vi "LogTracepoint.vi"(8 "error in (no error)":errorcluster, 9 "log string":string, 10 "tracepoint":string, 11 "qbus in":refnum<class "Qbus.lvclass">) -> (0 "error out":errorcluster, 3 "qbus out":refnum<class "Qbus.lvclass">)   [LabVIEW 2017, in "TraceLogger.lvlib"]
doc: "Writes an instance of a tracepoint to a temporary tracelog file on the device disk and sends the instance to NI InsightCM Server to be saved in its tracelog. If the tracepoint is disabled, this VI ignores the input."
uses:
  <vilib>/addons/TraceLogger/TraceLogger.lvlib
  <vilib>/addons/Qbus/Qbus.lvclass
  <vilib>/addons/TraceLogger/controls/LogTracepoint.ctl
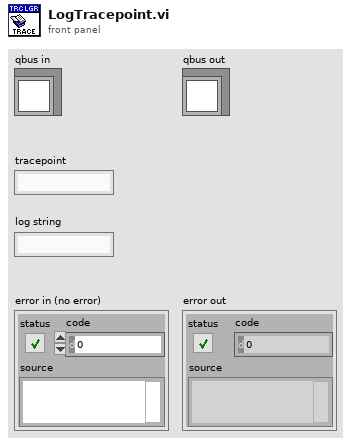
[diagram p1: front panel]
types:
  T1 = typedef "TraceLogger.lvlib/LogTracepoint.ctl" = cluster{"tracepoint":string, "log string":string}
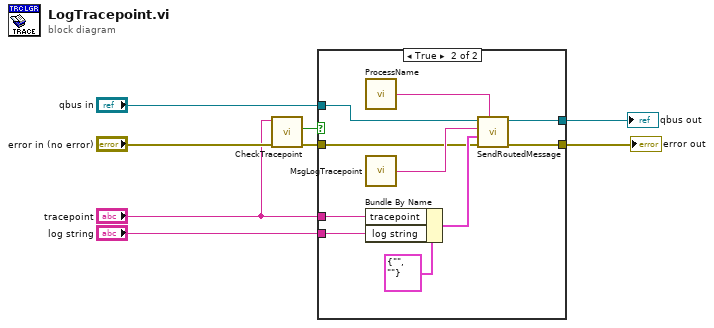
[diagram p0: block diagram]
diagram:
  n1 = call <vilib>:"CheckTracepoint.vi"("error in (no error)"="error in (no error)", "tracepoint"="tracepoint") -> ("error out"=w3:errorcluster, "enabled"=w1:bool)  [unwired: 7 in, 1 out]
  n2 = case shown="True" w1 {
    tunnel: "log string" -> [_ w18]
    tunnel: "qbus in" -> [w9 w16]
    tunnel: [w9 w14] -> w6
    tunnel: [w10 w13] -> w5
    tunnel: w3 -> [w10 w12]
    tunnel: "tracepoint" -> [_ w11]
    frame False {
    }
    frame True {
      n3 = call <vilib>:"ProcessName.vi"() -> ("process name"=w15:string)  [unwired: 5 in]
      n4 = call <vilib>:"MsgLogTracepoint.vi"() -> ("message name"=w20:string)  [unwired: 5 in]
      n5 = Bundle By Name(cluster=T1 {"tracepoint"="", "log string"=""} ("Tracelog"), "tracepoint"=w11, "log string"=w18) -> (w17:T1)
      n6 = call <vilib>:"SendRoutedMessage.vi"("listener process"=w15, "error in (no error)"=w12, "message value"=w17, "message name"=w20, "Qbus in"=w16) -> ("error in (no error)"=w13:errorcluster, "Qbus out"=w14:refnum<class "Qbus.lvclass">)  [unwired: 5 in]
    }
  }
  "qbus out" <- w6
  "error out" <- w5
